vi "Digital Read 1 Channel.vi"(8 "error in (no error)":errorcluster, 10 "Read":i32, 11 "NI-DAQ in":refnum<class "NI-DAQ.lvclass">) -> (0 "error out":errorcluster, 2 "Value":bool=TRUE, 3 "NI-DAQ out":refnum<class "NI-DAQ.lvclass">)   [LabVIEW 2020, in "NI-DAQ.lvclass"]
uses:
  NI-DAQ.lvclass
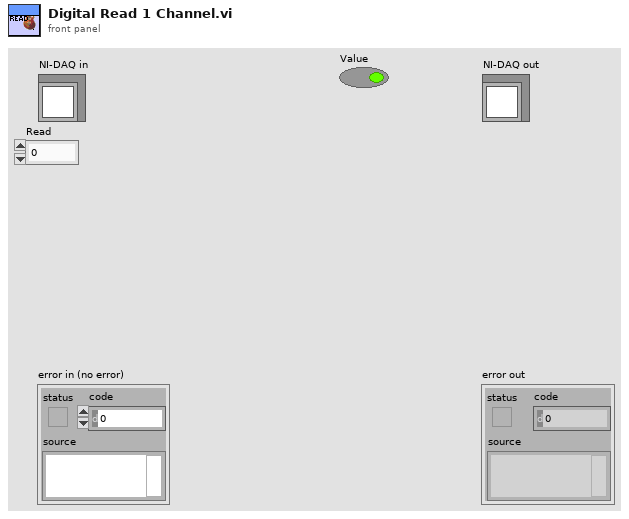
[diagram p1: front panel]
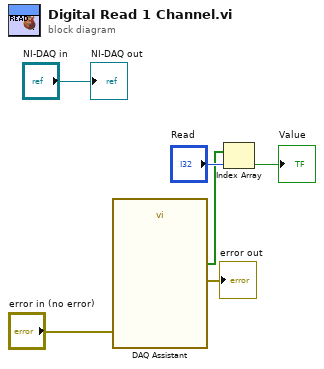
[diagram p0: block diagram]
diagram:
  n1 = call "DAQ Assistant"("error in"="error in (no error)") -> ("data"=w3:bool[], "error out"=→"error out":errorcluster)  [unwired: 16 in, 1 out]
  n2 = Index Array(array=w3, index="Read") -> (element=→"Value":bool)
  "NI-DAQ out" <- "NI-DAQ in"
